vi "Results Data.vi"() -> ()   [LabVIEW 2012]
panel:
  out "Waveform Chart":cluster{dbl, dbl, "HSSRPM (RPM)":sgl}[](graph)
  in  "History Data":cluster{dbl, dbl, "HSSRPM (RPM)":sgl}[](array[cluster])=array[400000 elements]
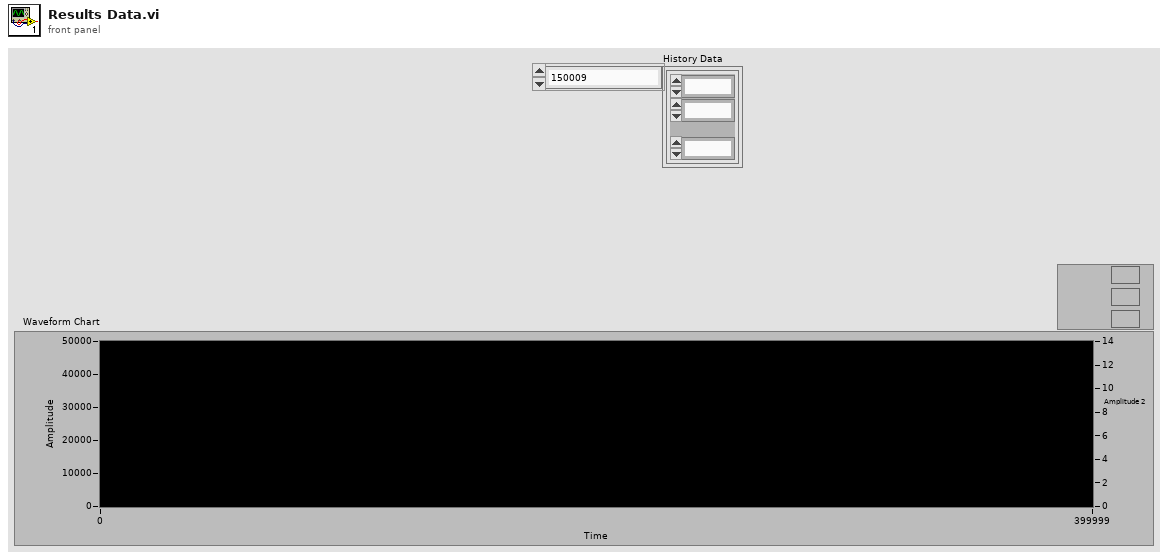
[diagram p1: front panel]
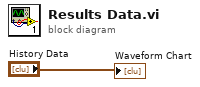
[diagram p0: block diagram]
diagram:
  "Waveform Chart" <- "History Data"
